vi "MU Set Interface.vi"(8 "error in (no error)":errorcluster, 9 "interfaceOption":string, 10 "interfaceType":u32, 11 "handle":u64) -> (0 "error out (no error)":errorcluster, 3 "function return":u32)   [LabVIEW 2017, in "MU_3SL_interface.lvlib"]
uses:
  MU_3SL_interface.lvlib
  lib/MU_3SL_interface.dll
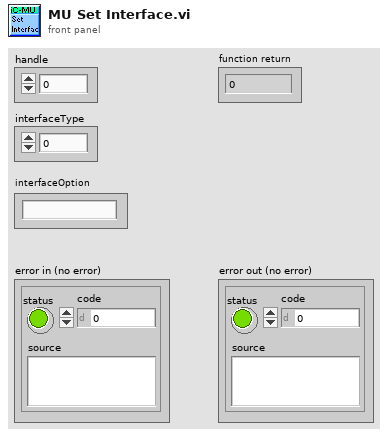
[diagram p1: front panel]
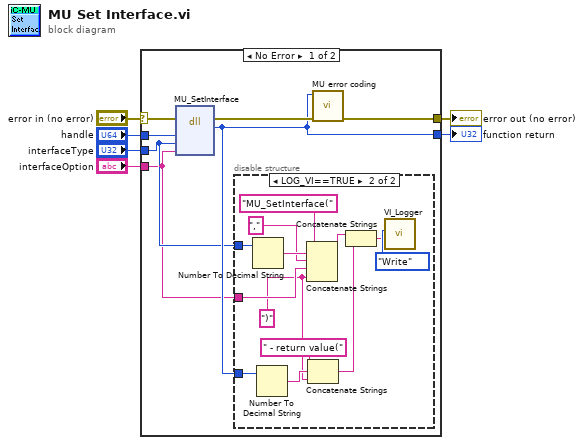
[diagram p0: block diagram]
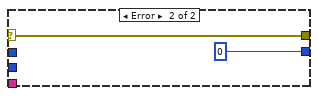
[diagram p3: hidden frame]
diagram:
  n1 = case shown="No Error" "error in (no error)" {
    selector: "error in (no error)" -> [w11 w28]
    tunnel: [w9 u32 0 ("return type")] -> w6
    tunnel: "handle" -> [w10 _]
    tunnel: "interfaceType" -> [w8 _]
    tunnel: "interfaceOption" -> [w7 _]
    tunnel: [w12 w28] -> w2
    frame No Error {
      n2 = dll-call lib="C:/Users/bes/AppData/Roaming/work/mu_9so/icsubmodules/soft_mu_3sl_master/lv_interface/lib/MU_3SL_interface**.*" fn="MU_SetInterface"(error in=w11, "handle"=w10, "interfaceType"=w8, "interfaceOption"=w7) -> (error out=w13:errorcluster, "return type"=w9:u32)  [unwired: 5 in, 1 out]
      n3 = disable-structure shown="LOG_VI==TRUE" {
        disable-tunnel: w9 -> [_ w24]
        disable-tunnel: w8 -> [_ w19]
        disable-tunnel: w7 -> [_ w16]
        frame condition #0 {
        }
        frame condition #1 (active) {
          w14 = ")" ("string")
          n4 = Number To Decimal String(number=w19) -> (decimal integer string=w18:string)  [unwired: 1 in]
          n5 = Number To Decimal String(number=w24) -> (decimal integer string=w23:string)  [unwired: 1 in]
          n6 = Concatenate Strings("MU_SetInterface(" ("Info in"), w18, "," ("string"), w16, w14) -> (w22:string)
          n7 = Concatenate Strings(" - return value(" ("string"), w23, w14) -> (w21:string)
          n8 = Concatenate Strings(w22, w21) -> (w20:string)
          n9 = call "VI_Logger.vi"("Action (Read)"=enum16{"Write", "Read"}."Write", "Info in"=w20) -> ()  [unwired: 8 in, 2 out]
        }
      }
      n10 = call "MU error coding.vi"("error in (no error)"=w13, "function return in"=w9) -> ("error out"=w12:errorcluster)  [unwired: 9 in]
    }
    frame Error {
    }
  }
  "function return" <- w6
  "error out (no error)" <- w2
